vi "startRun1.vi"(8 "error in":errorcluster, 9 "Boiler Simulation Controls":refnum<vi>, 10 "Boiler Controls":refnum<vi>, 11 "Boiler Status Indicators":refnum<vi>) -> (0 "error out":errorcluster)   [LabVIEW 2024]
uses:
  Controls/Boiler Simulation Controls.ctl
  Controls/Boiler Status Indicators.ctl
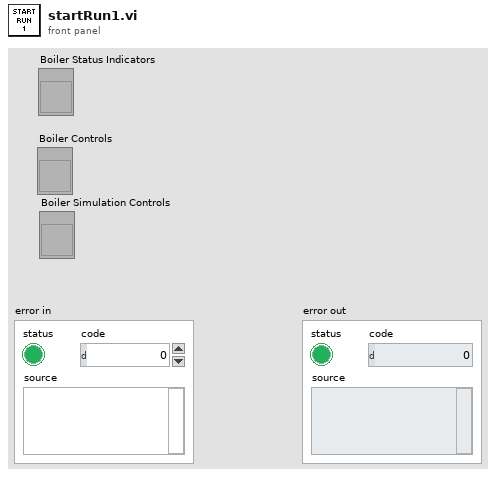
[diagram p1: front panel]
types:
  T1 = typedef "Boiler Status Indicators.ctl" = cluster{"Status":string, "Primary Fan":bool, "Natural Gas Valve":bool, "Pilot":bool, "Fuel Valve":bool, "Forced Draft Fan":bool, "Time Count":dbl}
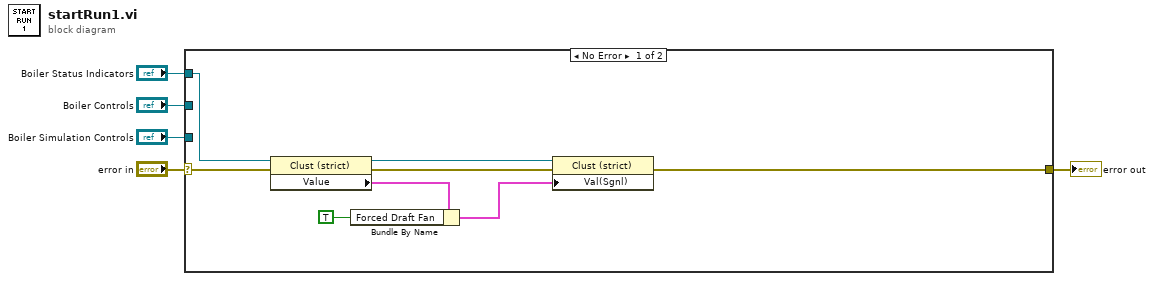
[diagram p0: block diagram]
diagram:
  n1 = case shown="No Error" "error in" {
    selector: "error in" -> [w13 w14]
    tunnel: [w7 w14] -> w4
    tunnel: "Boiler Status Indicators" -> [w6 _]
    tunnel: "Boiler Controls" -> [_ _]
    tunnel: "Boiler Simulation Controls" -> [_ _]
    frame No Error {
      n2 = property class="Clust (strict)"(reference=w6, error in=w13) -> (reference out=w10:refnum<vi>, error out=w9:errorcluster, "Value"=w12:T1)
      n3 = Bundle By Name(cluster=w12, "Forced Draft Fan"=TRUE) -> (w11:T1)
      n4 = property class="Clust (strict)"(reference=w10, error in=w9, "Val(Sgnl)"=w11) -> (error out=w7:errorcluster)  [unwired: 1 out]
    }
    frame Error {
    }
  }
  "error out" <- w4
